vi "Module ID.vi"(11 "Timing Module in":refnum<class "Timing Module.lvclass">) -> (2 "Module ID":string)   [LabVIEW 2020, in "Volatus.lvlib" / "Timing Module.lvclass"]
uses:
  Timing Module.lvclass
  Timing Module.lvclass/Timing Module.ctl
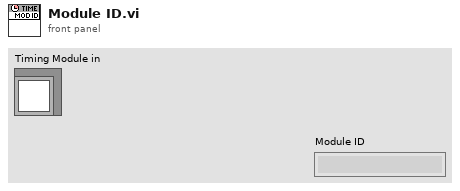
[diagram p1: front panel]
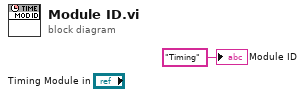
[diagram p0: block diagram]
diagram:
  "Module ID" <- "Timing" ("Module ID")
